vi "ReadConfigFile.vi"(8 "error in":errorcluster, 11 "ini file path in":path) -> (0 "error out":errorcluster, 2 "Sections/Keys/Values":T1(array[cluster]), 3 "ini file path out":path)   [LabVIEW 2013]
uses:
  <vilib>/Utility/config.llb/Read Key (String).vi
  <vilib>/Utility/config.llb/NI_LVConfig.lvlib
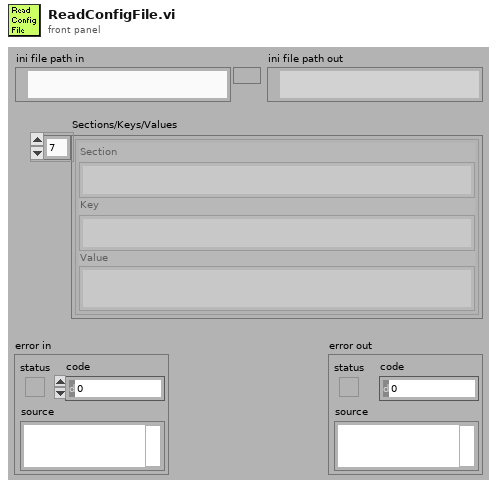
[diagram p1: front panel]
types:
  T1 = cluster{"Section":string, "Key":string, "Value":string}[]
  T2 = cluster{"Section":string, "Key":string, "Value":string}
  T3 = typedef "NI_LVConfig.lvlib/Config Data RefNum.ctl" = refnum<k1>
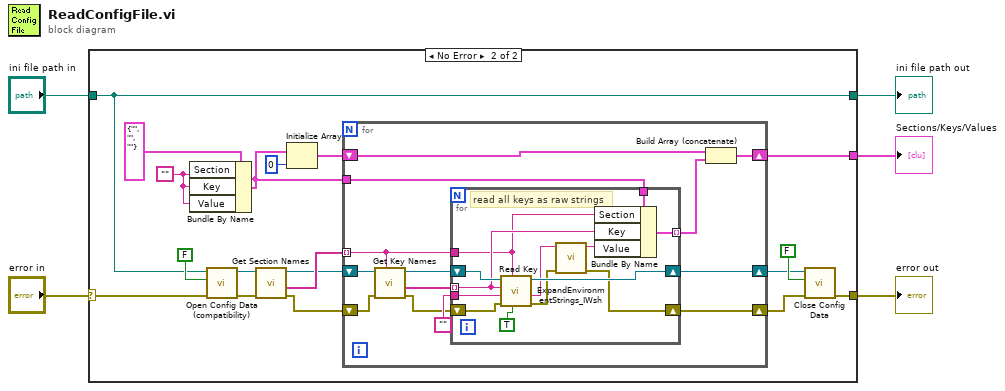
[diagram p0: block diagram]
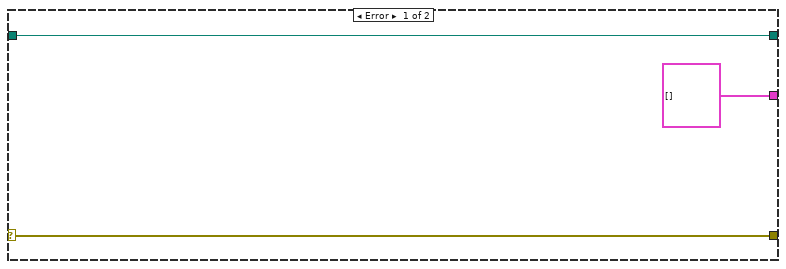
[diagram p2: hidden frame]
diagram:
  n1 = case shown="No Error" "error in" {
    selector: "error in" -> [w6 w10]
    tunnel: [w6 w26] -> w5
    tunnel: [T1 [] w14] -> w4
    tunnel: "ini file path in" -> [w8 w11]
    tunnel: [w8 w11] -> w1
    frame Error {
    }
    frame No Error {
      w12 = ""
      n2 = Bundle By Name(cluster=T2 {"Section"="", "Key"="", "Value"=""} ("Key/Value"), "Section"=w12, "Key"=w12, "Value"=w12) -> (w16:T2)
      n3 = call <vilib>:"Open Config Data (compatibility).vi"("error in (no error)"=w10, "create file if necessary (T)"=FALSE ("create file if necessary? (T)"), "configuration file path"=w11) -> ("error out"=w22:errorcluster, "refnum"=w23:T3)  [unwired: 6 in, 1 out]
      n4 = call <vilib>:"Get Section Names.vi"("error in (no error)"=w22, "refnum"=w23) -> ("error out"=w18:errorcluster, "section names"=w20:string[], "refnum out"=w19:T3)  [unwired: 7 in]
      n5 = Initialize Array(w16, 0 ("dimension size")) -> (w15:T1)
      n6 = for {
        tunnel: w20 -> [w33] mode=indexing
        shift-right: [w35] -> w14
        shift-left: w15 -> [w36]
        tunnel: w16 -> [w28]
        shift-right: [w38] -> w24
        shift-left: w19 -> [w31]
        shift-right: [w27] -> w9
        shift-left: w18 -> [w32]
        n7 = call <vilib>:"Get Key Names.vi"("section"=w33, "error in (no error)"=w32, "refnum"=w31) -> ("error out"=w29:errorcluster, "key names"=w34:string[], "refnum out"=w30:T3)  [unwired: 5 in, 1 out]
        n8 = for {
          tunnel: w34 -> [w47] mode=indexing
          tunnel: "" ("default value") -> [w50]
          tunnel: [w48] -> w37 mode=indexing
          shift-right: [w49] -> w38
          shift-left: w30 -> [w51]
          tunnel: w33 -> [w45]
          tunnel: w28 -> [w46]
          shift-right: [w42] -> w27
          shift-left: w29 -> [w52]
          # "read all keys as raw strings"
          n9 = call-poly <vilib>:"Read Key.vi"("read raw string? (F)"=TRUE, "section"=w45, "error in (no error)"=w52, "default value"=w50, "key"=w47, "refnum"=w51) -> ("error out"=w43:errorcluster, "value"=w41:string, "refnum out"=w49:T3)  [unwired: 2 in, 1 out]
          n10 = call "ExpandEnvironmentStrings_IWsh.vi"("error in (no error)"=w43, "String w/ \nEnvironment Variable(s)"=w41) -> ("error out"=w42:errorcluster, "Expanded String"=w44:string)  [unwired: 5 in, 1 out]
          n11 = Bundle By Name(cluster=w46, "Section"=w45, "Key"=w47, "Value"=w44) -> (w48:T2)
        }
        n12 = Build Array (concatenate)(w36, w37) -> (w35:T1)
      }
      n13 = call <vilib>:"Close Config Data.vi"("error in (no error)"=w9, "write file if changed (T)"=FALSE ("write configuration file? (T)"), "refnum"=w24) -> ("error out"=w26:errorcluster)  [unwired: 7 in, 1 out]
    }
  }
  "error out" <- w5
  "Sections/Keys/Values" <- w4
  "ini file path out" <- w1
